vi "GlobalGetCamerasOnOff.vi"() -> ()   [LabVIEW 2009]
panel:
  in  "cam2":bool
  in  "cam1":bool
  out "GetCamera":bool
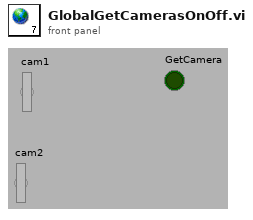
[diagram p1: front panel]
diagram:
